vi "_CleanUpThread.vi"(10 "SyncUpQueue":refnum<queue>, 11 "ReturnQUEUE":refnum<queue>) -> ()   [LabVIEW 2017, in "MDPtr.lvlib" / "MDPtrMgr.lvclass"]
uses:
  MDPtrMgr.lvclass
  Def-Request.ctl
  Def-Respone.ctl
  MDPtr TypeDef/MDPtr DataFrame-Memory.ctl
  MDPtr TypeDef/MDPtr DataFrame-Common.ctl
  <vilib>/Utility/Data Type/Type Definitions/Data Type.ctl
  MDPtr TypeDef/MDPtr Queue.ctl
  MDPtr TypeDef/MDPtr.ctl
  MDPtr.lvlib
  <vilib>/Utility/Data Type/NI_Data Type.lvlib
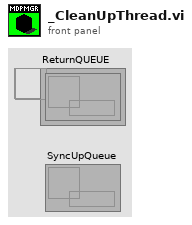
[diagram p1: front panel]
types:
  T1 = typedef "MDPtr.lvlib/Def-Respone.ctl" = cluster{"MDPtr DVR":refnum<data-value>, "error out":errorcluster, "MDPtrQueue":T2}
  T2 = typedef "MDPtr.lvlib/MDPtr Queue.ctl" = refnum<queue>
  T3 = typedef "MDPtr.lvlib/MDPtr.ctl" = refnum<k1>
  T4 = typedef "MDPtr.lvlib/Def-Request.ctl" = cluster{"Type":enum16{"DVR", "Queue"}, "Cache Length":i32, "ResponeQueue":refnum<queue>}
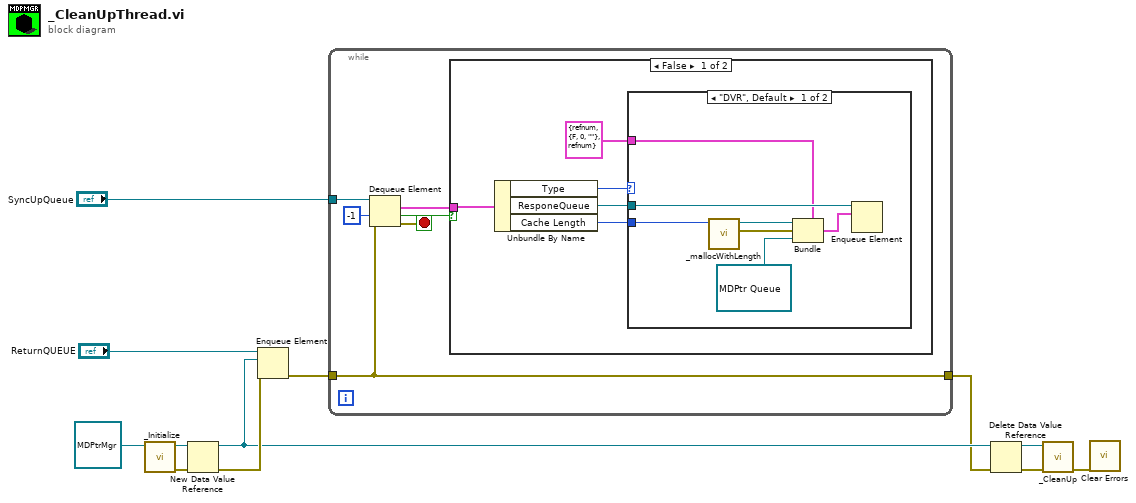
[diagram p0: block diagram]
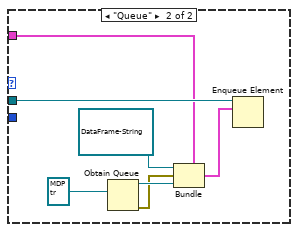
[diagram p2: hidden frame]
diagram:
  n1 = call "_Initialize.vi"("MDPtrMgr in"=refnum<class "MDPtrMgr.lvclass"> refnum) -> ("error out"=w11:errorcluster, "MDPtrMgr out"=w10:refnum<class "MDPtrMgr.lvclass">)  [unwired: 9 in]
  n2 = New Data Value Reference(data value=w10, error in=w11) -> (data value reference=w6:refnum<data-value>, error out=w7:errorcluster)
  n3 = Enqueue Element(queue="ReturnQUEUE", element=w6, error in (no error)=w7) -> (error out=w8:errorcluster)  [unwired: 1 in, 2 out]
  n4 = while {
    tunnel: "SyncUpQueue" -> [w17]
    tunnel: w8 -> [w15]
    tunnel: [w15] -> w5
    stop <- w16 stop-if-true
    n5 = Dequeue Element(queue=w17, timeout in ms (-1)=-1, error in (no error)=w15) -> (element=w13:T4, timed out?=w14:bool, error out=w16:errorcluster)  [unwired: 1 out]
    n6 = case shown="False" w14 {
      tunnel: w13 -> [w23 _]
      frame False {
        n7 = Unbundle By Name(w23) -> ("Type"=w20:enum16{"DVR", "Queue"}, "ResponeQueue"=w21:refnum<queue>, "Cache Length"=w22:i32)
        n8 = case shown="\"DVR\", Default" w20 {
          tunnel: w22 -> [w30 _]
          tunnel: w21 -> [w29 w37]
          tunnel: T1 {"MDPtr DVR"=refnum, "error out"={"status"=FALSE, "code"=0, "source"=""}, "MDPtrQueue"=refnum} ("Request") -> [w28 w36]
          frame "DVR", Default {
            n9 = call "_mallocWithLength.vi"("Common.Data Length"=w30) -> ("error out"=w26:errorcluster, "MDPtr DVR"=w27:refnum<data-value>)  [unwired: 9 in]
            n10 = Bundle(cluster=w28, "MDPtr DVR"=w27, "error out"=w26, "MDPtrQueue"=T2 refnum) -> (w24:T1)
            n11 = Enqueue Element(queue=w29, element=w24) -> ()  [unwired: 2 in, 3 out]
          }
          frame "Queue" {
            n12 = Obtain Queue(element data type=T3 refnum ("MDPtr")) -> (queue out=w33:refnum<queue>, error out=w31:errorcluster)  [unwired: 4 in, 1 out]
            n13 = Bundle(cluster=w36, "MDPtr DVR"=refnum<data-value> refnum, "error out"=w31, "MDPtrQueue"=w33) -> (w35:T1)
            n14 = Enqueue Element(queue=w37, element=w35) -> ()  [unwired: 2 in, 3 out]
          }
        }
      }
      frame True {
      }
    }
  }
  n15 = Delete Data Value Reference(data value reference=w6, error in=w5) -> (data value=w3:refnum<class "MDPtrMgr.lvclass">, error out=w4:errorcluster)
  n16 = call "_CleanUp.vi"("error in (no error)"=w4, "MDPtrMgr in"=w3) -> ("error out"=w2:errorcluster)  [unwired: 8 in, 1 out]
  n17 = call <vilib>:"Clear Errors.vi"("error in (no error)"=w2) -> ()  [unwired: 5 in, 2 out]
